vi "HXG2_dTchecker.vi"(10 "error in (no error)":errorcluster, 11 "Previous":dbl) -> (2 "error out":errorcluster, 3 "Previous Time":dbl, 5 "dT":dbl)   [LabVIEW 2010]
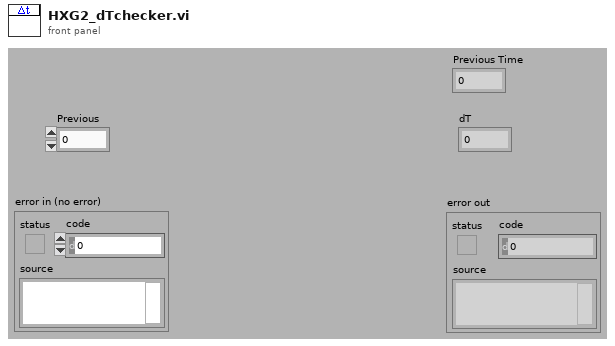
[diagram p1: front panel]
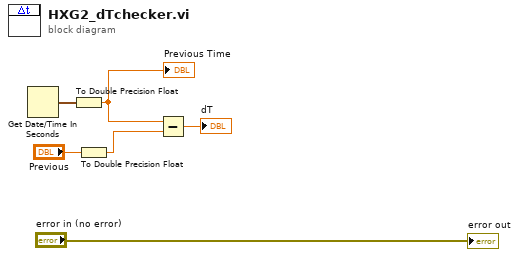
[diagram p0: block diagram]
diagram:
  n1 = Get Date/Time In Seconds() -> (seconds since 1Jan1904=w6:timestamp)
  n2 = To Double Precision Float(number=w6) -> (double precision float=w5:dbl)
  "Previous Time" <- w5
  n3 = To Double Precision Float(number="Previous") -> (double precision float=w4:dbl)
  n4 = Subtract(x=w5, y=w4) -> (x-y=→"dT":dbl)
  "error out" <- "error in (no error)"
